vi "SourceDialog.vi"(8 "Error In":errorcluster, 11 "Source Configurations In":T1[](array[typedef])) -> (0 "Error Out":errorcluster, 2 "Cancelled?":bool, 3 "Source Configurations Out":T1[](array[typedef]))   [LabVIEW 2012]
uses:
  SourceConfiguration.ctl
  SourceFunction.ctl
  libs/LV-Utilities/LV-Utilities.lvlib
panel:
  in  "SMU B Auto Range Active?":bool=TRUE
  in  "SMU B Low Limit (V or A)":dbl format="%_4p"
  in  "SMU B High Limit (V or A)":dbl format="%_4p"
  in  "SMU B Active?":bool=TRUE
  in  "SMU B Level (V or A)":dbl format="%_4p"
  in  "SMU B Function":enum16{"Voltage", "Current"}(ring)
  in  "SMU A Auto Range Active?":bool=TRUE
  in  "SMU A Low Limit (V or A)":dbl format="%_4p"
  in  "SMU A High Limit (V or A)":dbl format="%_4p"
  in  "SMU A Active?":bool=TRUE
  in  "SMU A Level (V or A)":dbl format="%_4p"
  in  "SMU A Function":enum16{"Voltage", "Current"}(ring)
  in  "CANCEL":bool
  in  "DONE":bool
  # "SOURCE-MEASURE UNIT B"
  # "Range"
  # "Auto"
  # "Low Limit"
  # "High Limit"
  # "General"
  # "Active"
  # "Level"
  # "Function"
  # "SOURCE-MEASURE UNIT A"
  # "Range"
  # "Auto"
  # "Low Limit"
  # "High Limit"
  # "General"
  # "Active"
  # "Level"
  # "Function"
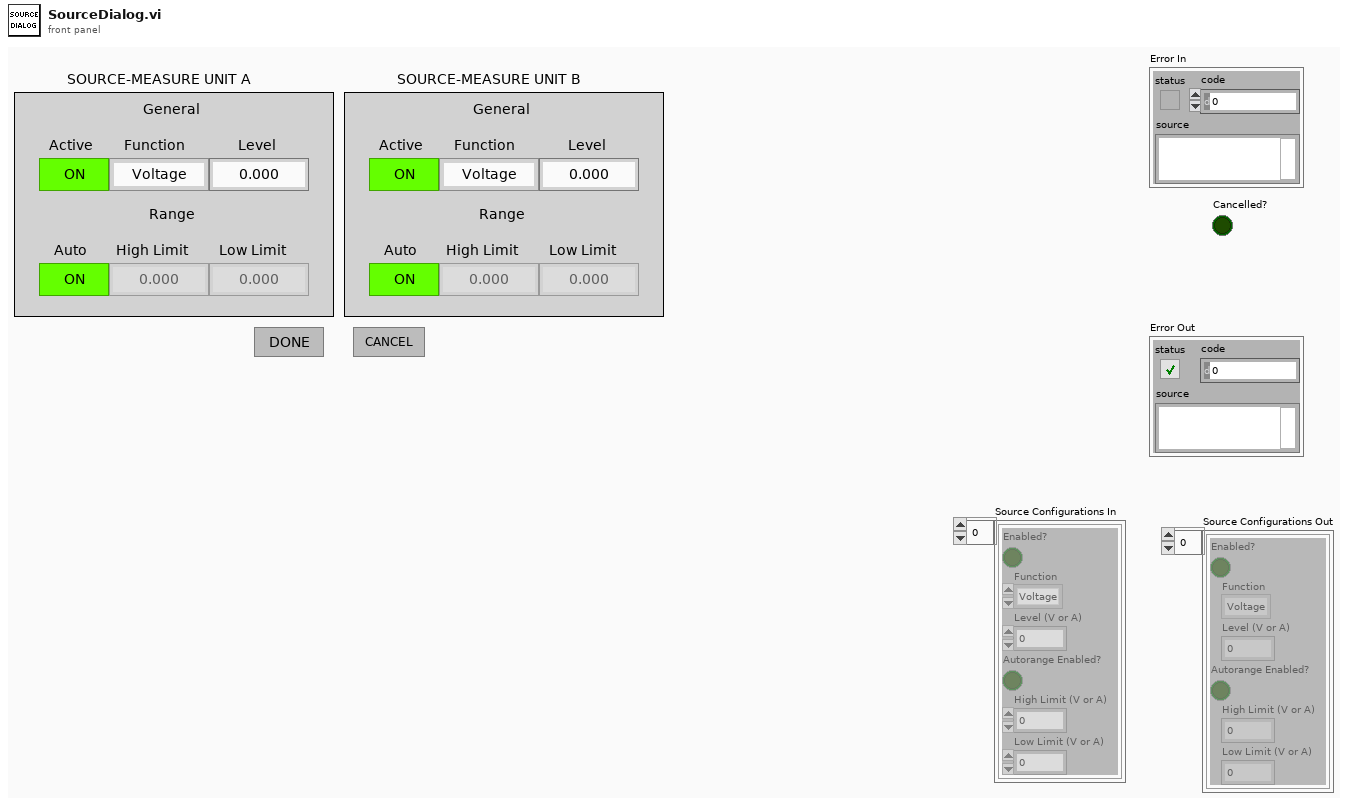
[diagram p1: front panel]
types:
  T1 = typedef "SourceConfiguration.ctl" = cluster{"Enabled?":bool, "Function":T2, "Level (V or A)":dbl, "Autorange Enabled?":bool, "High Limit (V or A)":dbl, "Low Limit (V or A)":dbl}
  T2 = typedef "SourceFunction.ctl" = enum16{"Voltage", "Current"}
  T3 = enum8{"Enabled", "Disabled", "Disabled and Grayed Out"}
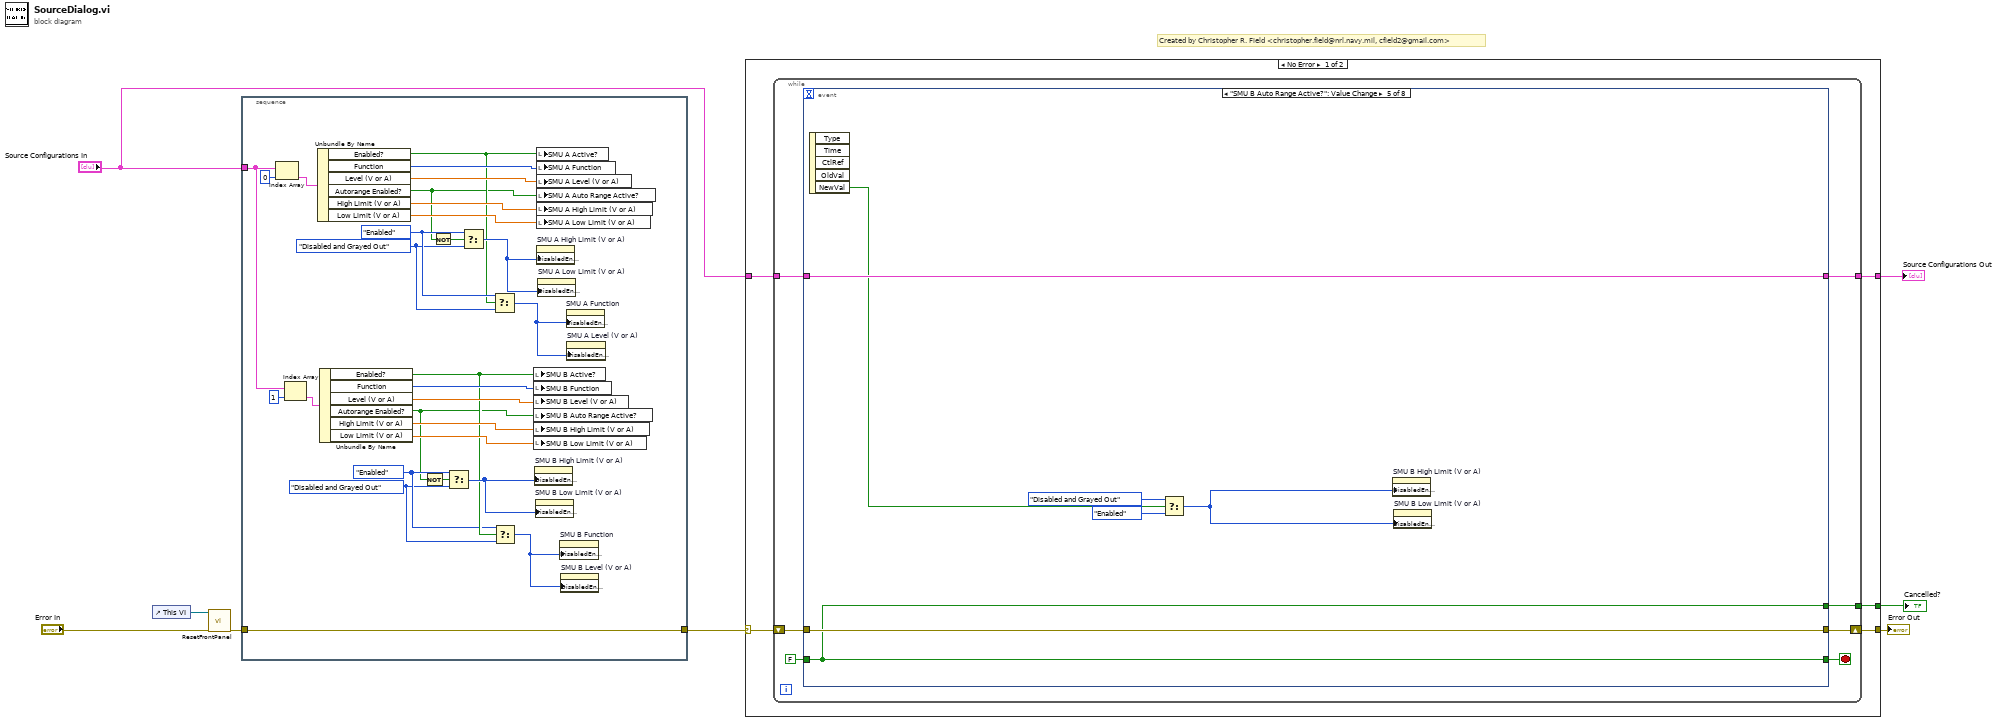
[diagram p0: block diagram]
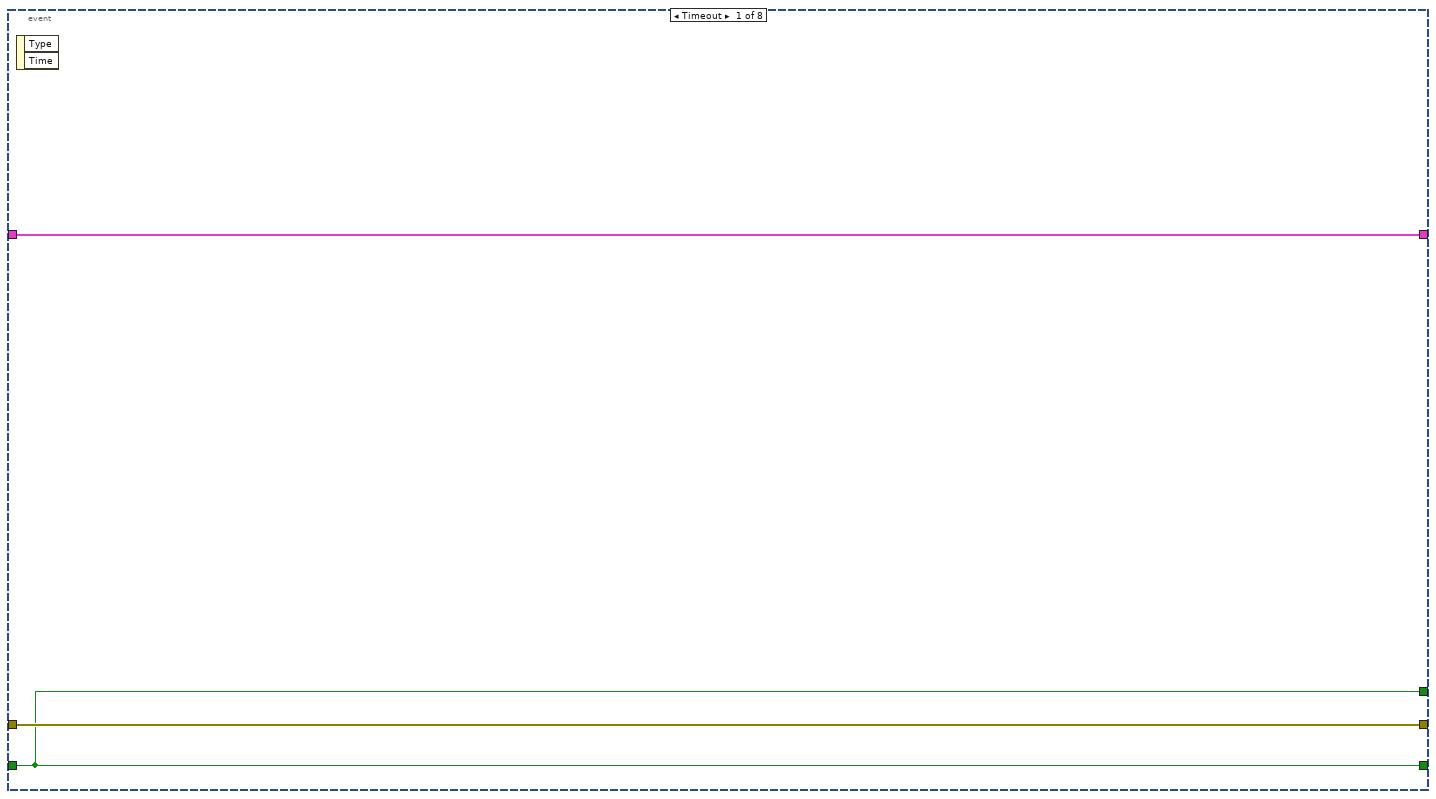
[diagram p2: hidden frame]
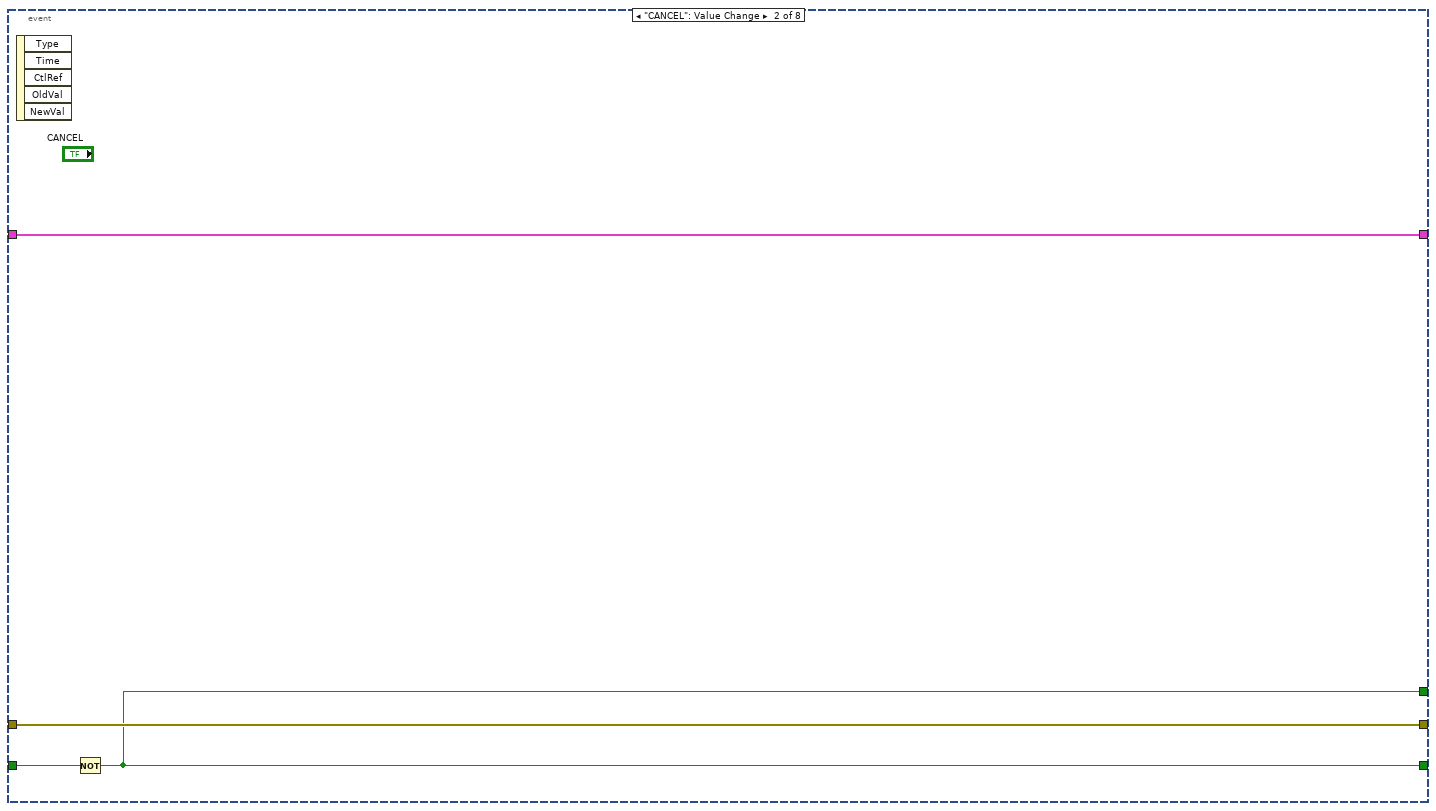
[diagram p3: hidden frame]
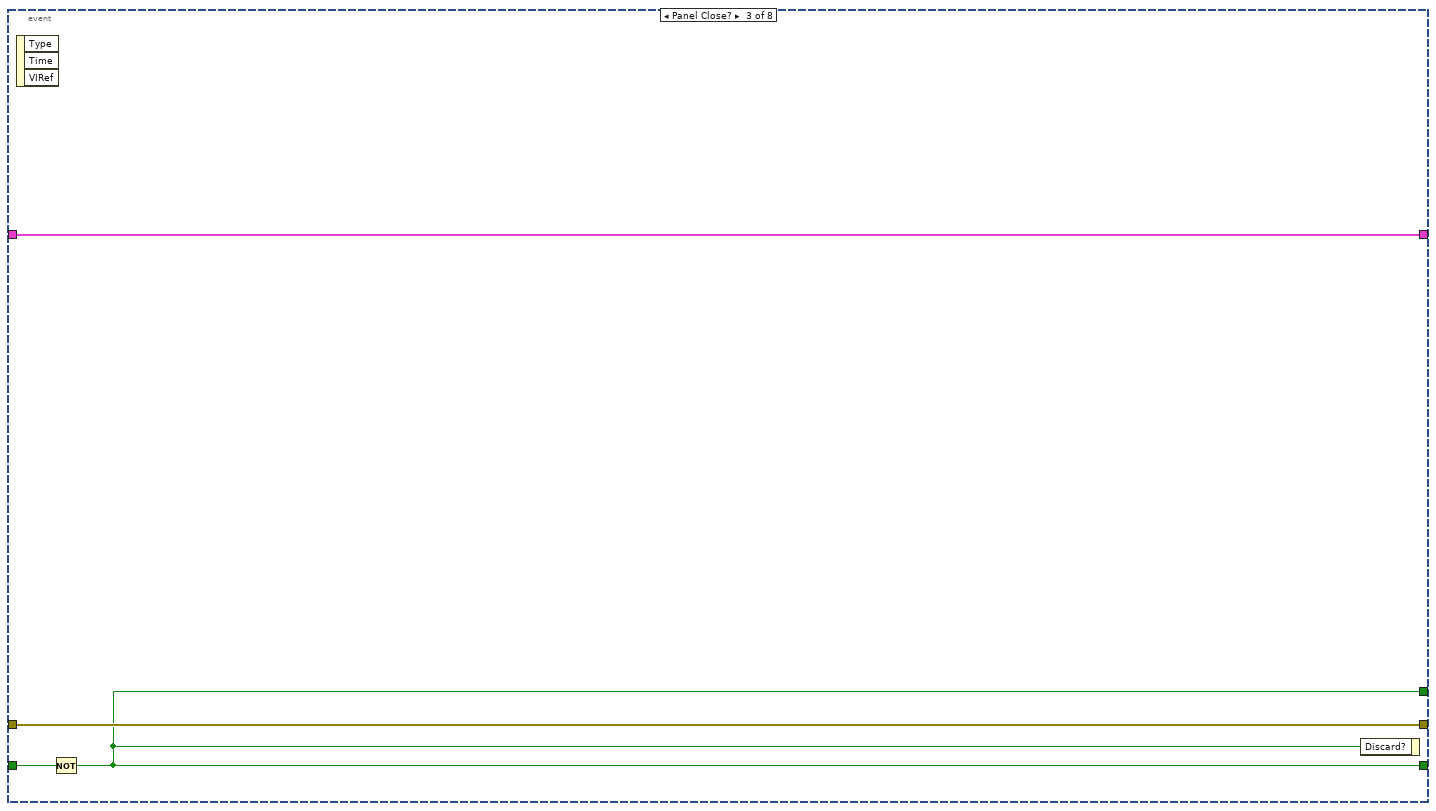
[diagram p4: hidden frame]
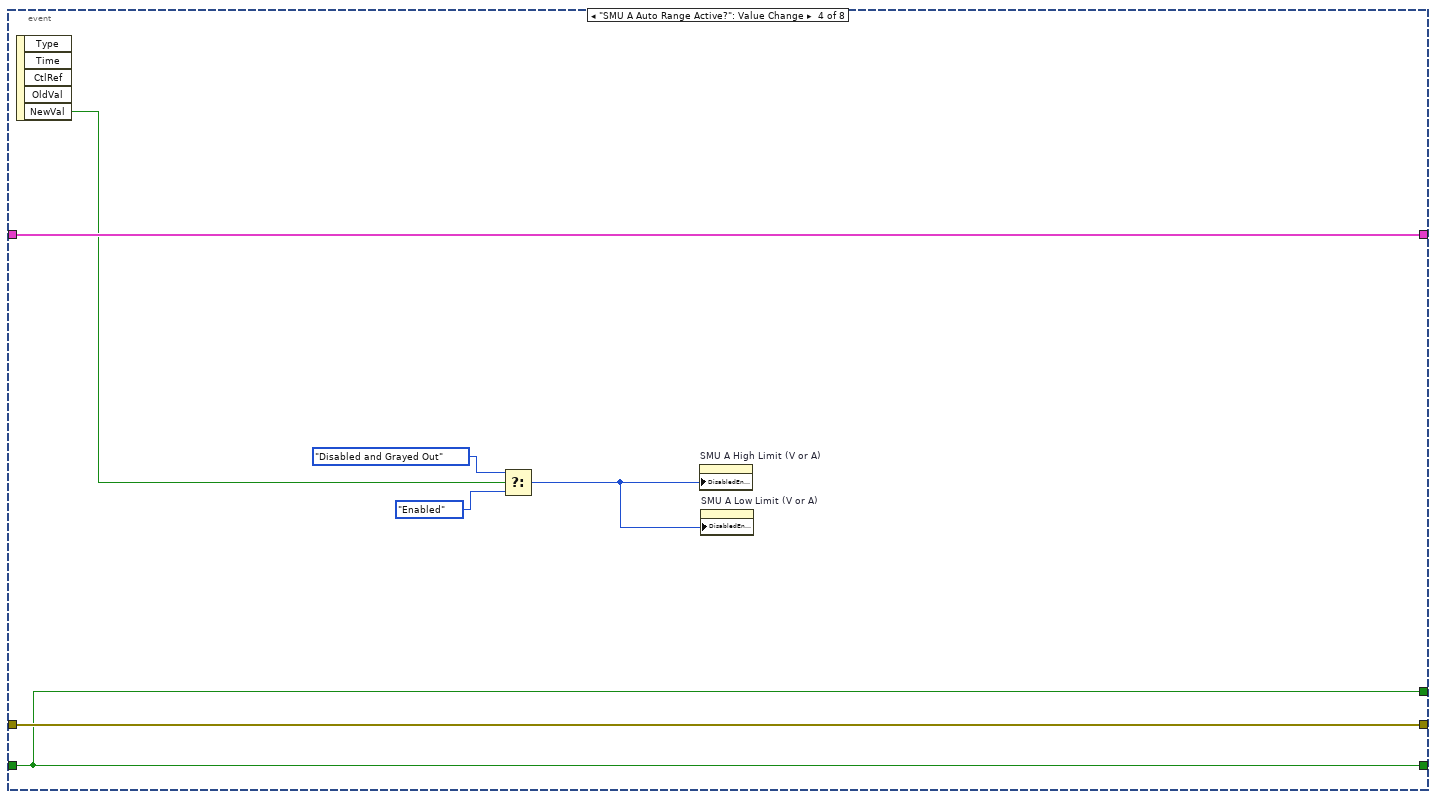
[diagram p5: hidden frame]
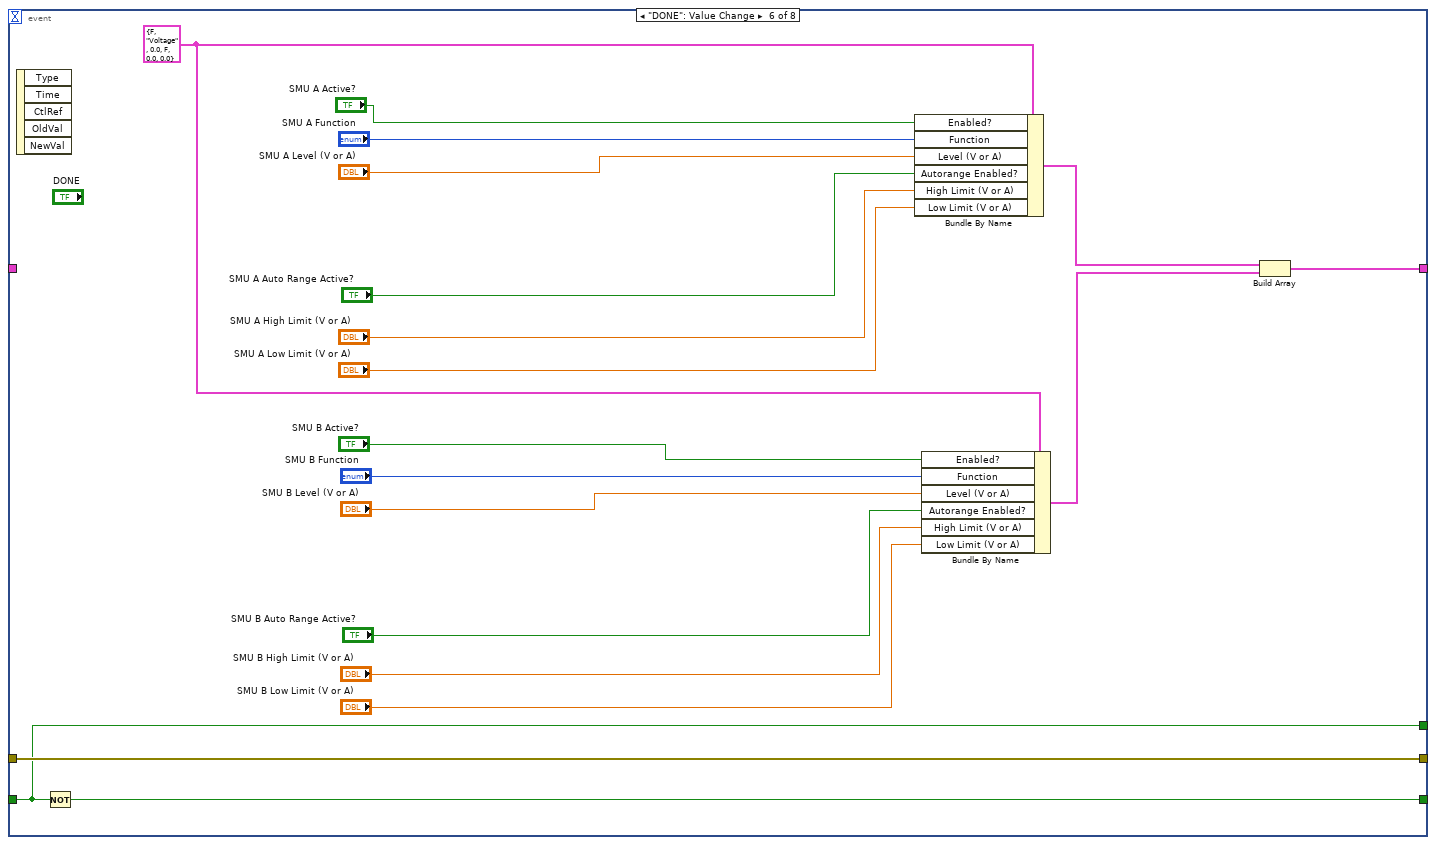
[diagram p6: hidden frame]
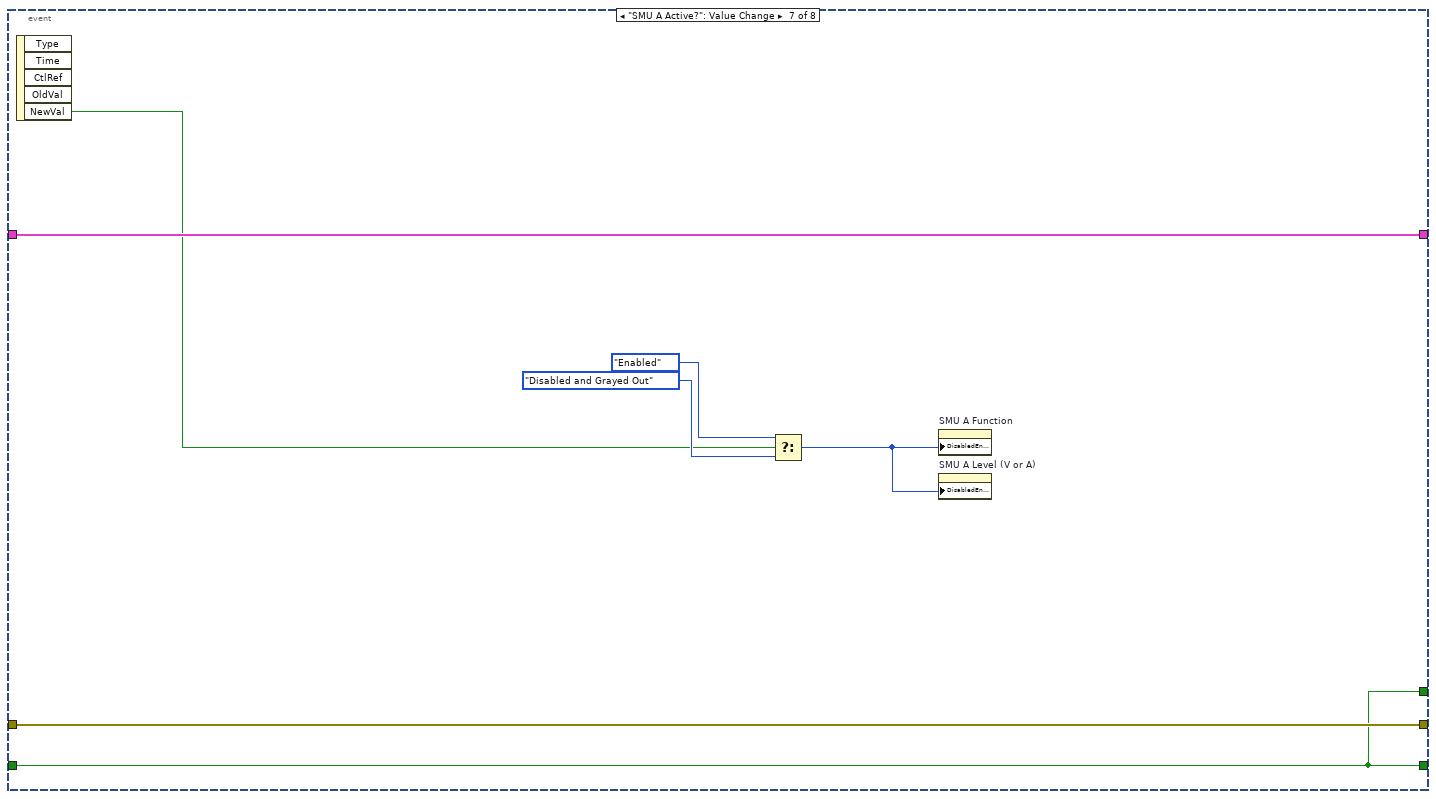
[diagram p7: hidden frame]
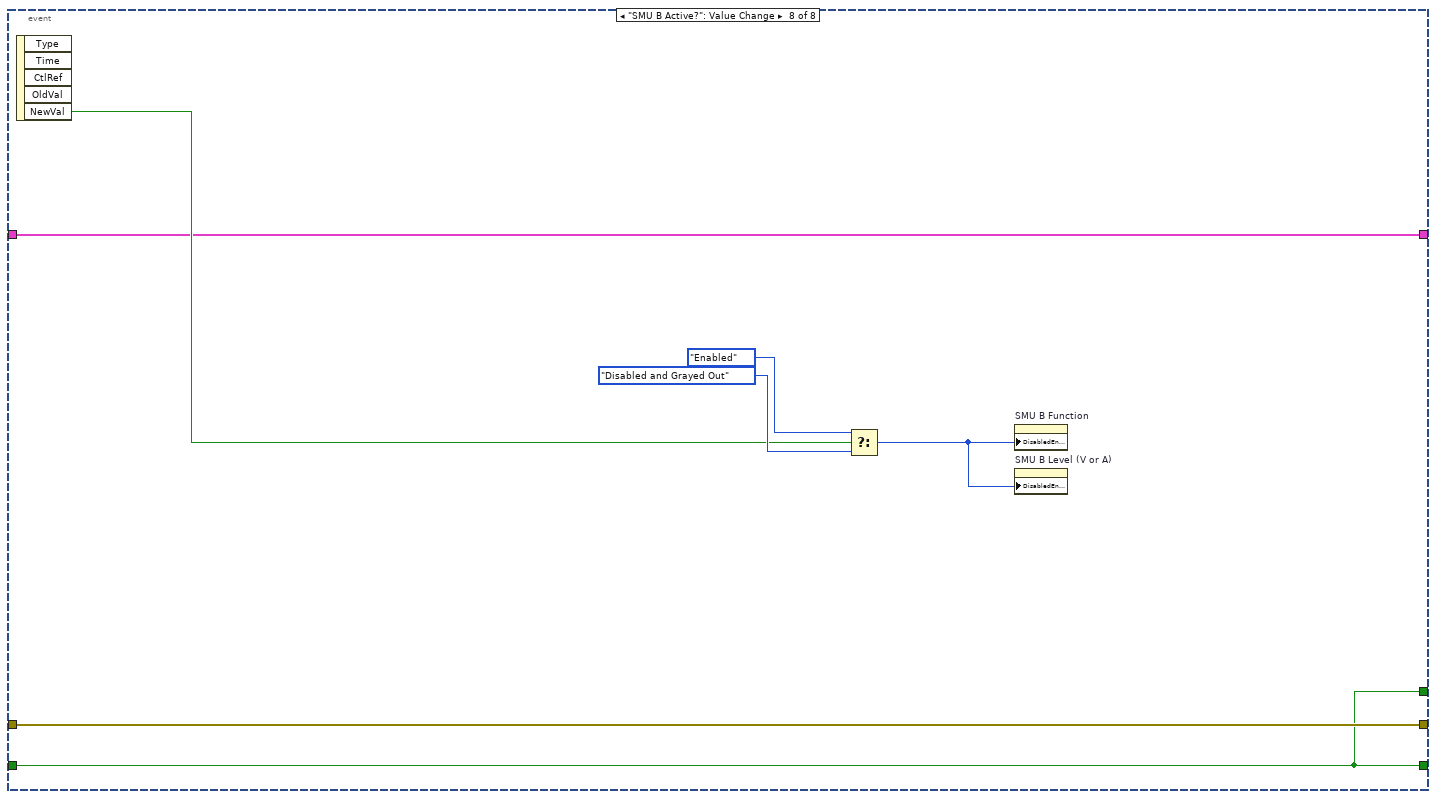
[diagram p8: hidden frame]
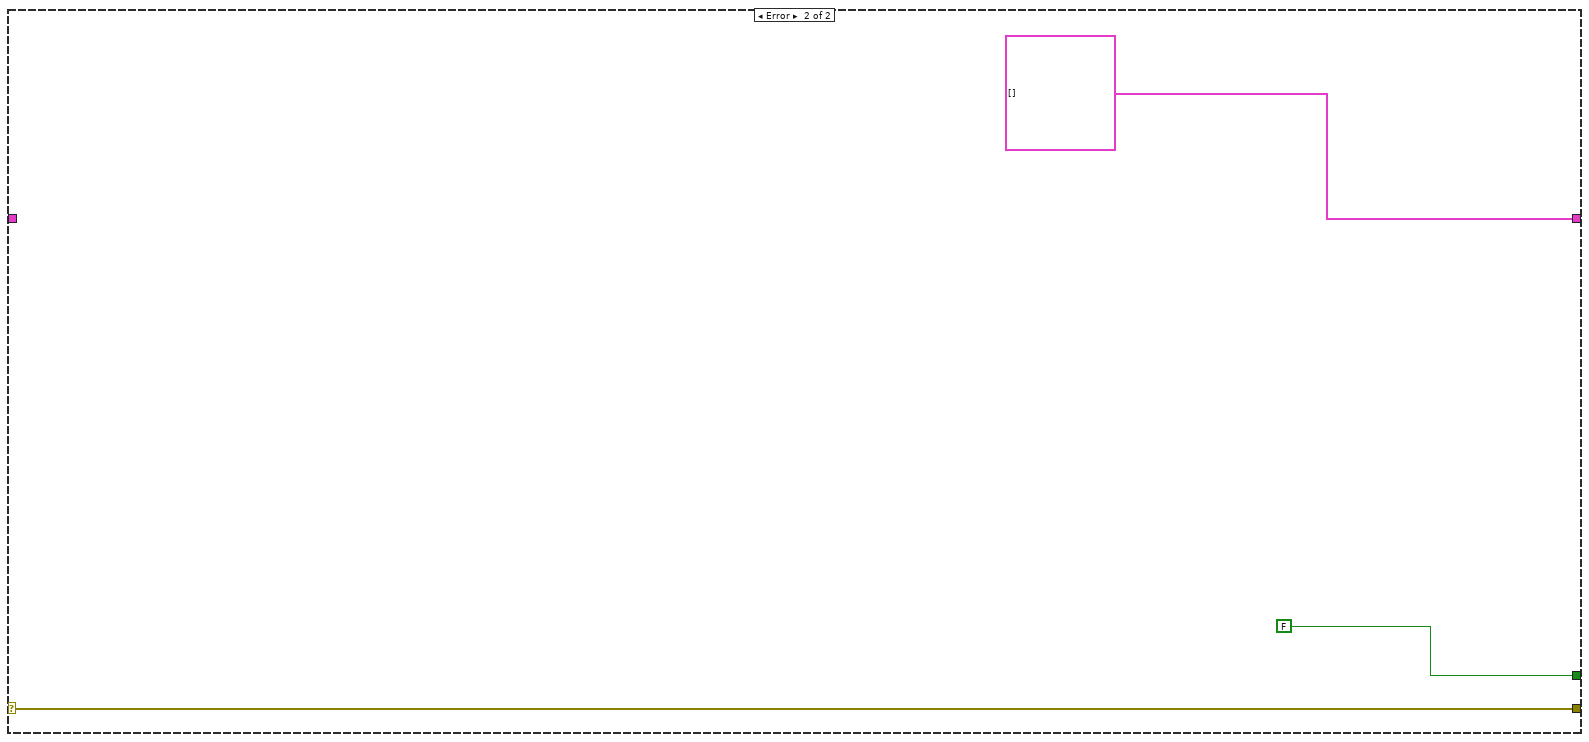
[diagram p9: hidden frame]
diagram:
  # "Created by Christopher R. Field <christopher.field@nrl.navy.mil, cfield2@gmail.com>"
  n1 = control-ref of="This VI"() -> (w1:refnum<vi>)
  n2 = call "ResetFrontPanel.vi"("Error In"="Error In", "VI Ref In"=w1) -> ("Error Out"=w4:errorcluster)  [unwired: 8 in, 1 out]
  n3 = stacked-sequence {
    tunnel: w4 -> [w36]
    tunnel: [w36] -> w3
    tunnel: "Source Configurations In" -> [w29]
    frame #0 {
      w18 = T3."Disabled and Grayed Out" ("f")
      w19 = T3."Enabled" ("Disabled")
      w13 = T3."Disabled and Grayed Out" ("f")
      w14 = T3."Enabled" ("Disabled")
      n4 = Index Array(array=w29, index=0) -> (element=w34:T1)
      n5 = Index Array(array=w29, index=1) -> (element=w27:T1)
      n6 = Unbundle By Name(w34) -> ("Enabled?"=w17:bool, "Function"=w33:T2, "Level (V or A)"=w32:dbl, "Autorange Enabled?"=w9:bool, "High Limit (V or A)"=w31:dbl, "Low Limit (V or A)"=w30:dbl)
      n7 = Unbundle By Name(w27) -> ("Enabled?"=w15:bool, "Function"=w26:T2, "Level (V or A)"=w25:dbl, "Autorange Enabled?"=w12:bool, "High Limit (V or A)"=w24:dbl, "Low Limit (V or A)"=w23:dbl)
      n8 = Not(x=w12) -> (.not. x?=w11:bool)
      n9 = Not(x=w9) -> (.not. x?=w10:bool)
      n10 = Select(t=w14, s=w11, f=w13) -> (s? t:f=w22:T3)
      n11 = Select(t=w19, s=w10, f=w18) -> (s? t:f=w21:T3)
      n12 = Select(t=w19, s=w17, f=w18) -> (s? t:f=w20:T3)
      n13 = Select(t=w14, s=w15, f=w13) -> (s? t:f=w16:T3)
      n14 = local write "SMU B Active?"(w15) -> ()
      n15 = local write "SMU B Function"(w26) -> ()
      n16 = local write "SMU B Level (V or A)"(w25) -> ()
      n17 = local write "SMU B Auto Range Active?"(w12) -> ()
      n18 = local write "SMU B High Limit (V or A)"(w24) -> ()
      n19 = local write "SMU B Low Limit (V or A)"(w23) -> ()
      n20 = property on="SMU B High Limit (V or A)" class="DigNum (strict)"("DisabledEnum"=w22) -> ()  [unwired: 2 in, 2 out]
      n21 = property on="SMU B Low Limit (V or A)" class="DigNum (strict)"("DisabledEnum"=w22) -> ()  [unwired: 2 in, 2 out]
      n22 = local write "SMU A Active?"(w17) -> ()
      n23 = local write "SMU A Function"(w33) -> ()
      n24 = local write "SMU A Level (V or A)"(w32) -> ()
      n25 = local write "SMU A Auto Range Active?"(w9) -> ()
      n26 = local write "SMU A High Limit (V or A)"(w31) -> ()
      n27 = local write "SMU A Low Limit (V or A)"(w30) -> ()
      n28 = property on="SMU A High Limit (V or A)" class="DigNum (strict)"("DisabledEnum"=w21) -> ()  [unwired: 2 in, 2 out]
      n29 = property on="SMU A Low Limit (V or A)" class="DigNum (strict)"("DisabledEnum"=w21) -> ()  [unwired: 2 in, 2 out]
      n30 = property on="SMU B Function" class="Enum (strict)"("DisabledEnum"=w16) -> ()  [unwired: 2 in, 2 out]
      n31 = property on="SMU B Level (V or A)" class="DigNum (strict)"("DisabledEnum"=w16) -> ()  [unwired: 2 in, 2 out]
      n32 = property on="SMU A Function" class="Enum (strict)"("DisabledEnum"=w20) -> ()  [unwired: 2 in, 2 out]
      n33 = property on="SMU A Level (V or A)" class="DigNum (strict)"("DisabledEnum"=w20) -> ()  [unwired: 2 in, 2 out]
    }
  }
  n34 = case shown="No Error" w3 {
    selector: w3 -> [w40 w109]
    tunnel: [w41 w109] -> w7
    tunnel: [w39 FALSE] -> w6
    tunnel: [w38 T1[] []] -> w5
    tunnel: "Source Configurations In" -> [w37 _]
    frame No Error {
      n35 = while {
        shift-right: [w46] -> w41
        shift-left: w40 -> [w45]
        tunnel: [w44] -> w39
        tunnel: [w43] -> w38
        tunnel: w37 -> [w42]
        stop <- w47 stop-if-true
        n36 = event shown="[4] \"SMU B Auto Range Active?\": Value Change" {
          selector: _ -> [_ _ _ _ _ _ _ _]
          dyn-events: _ -> [_ _ _ _ _ _ _ _]
          timeout: _ -> [_ _ _ _ _ _ _ _]
          tunnel: FALSE -> [w50 w55 w59 w65 w72 w90 w97 w100]
          tunnel: [w50 w53 w57 w65 w72 w92 w97 w100] -> w47
          tunnel: w45 -> [w51 w54 w58 w66 w73 w91 w98 w101]
          tunnel: [w51 w54 w58 w66 w73 w91 w98 w101] -> w46
          tunnel: [w50 w53 w57 w65 w72 w90 w97 w100] -> w44
          tunnel: [w49 w52 w56 w64 w71 w78 w99 w102] -> w43
          tunnel: w42 -> [w49 w52 w56 w64 w71 _ w99 w102]
          event Timeout {
            n37 = event-data() -> ()  [unwired: 1 in, 2 out]
          }
          event "CANCEL": Value Change {
            n38 = event-data() -> ()  [unwired: 1 in, 5 out]
            n39 = Not(x=w55) -> (.not. x?=w53:bool)
          }
          event Panel Close? {
            n40 = event-data() -> ()  [unwired: 1 in, 3 out]
            n41 = Not(x=w59) -> (.not. x?=w57:bool)
            n42 = event-data("Discard?"=w57) -> ()  [unwired: 1 in, 1 out]
          }
          event "SMU A Auto Range Active?": Value Change {
            n43 = event-data() -> ("NewVal"=w63:bool)  [unwired: 1 in, 4 out]
            n44 = Select(t=T3."Disabled and Grayed Out" ("Disabled"), s=w63, f=T3."Enabled" ("Disabled")) -> (s? t:f=w60:T3)
            n45 = property on="SMU A High Limit (V or A)" class="DigNum (strict)"("DisabledEnum"=w60) -> ()  [unwired: 2 in, 2 out]
            n46 = property on="SMU A Low Limit (V or A)" class="DigNum (strict)"("DisabledEnum"=w60) -> ()  [unwired: 2 in, 2 out]
          }
          event "SMU B Auto Range Active?": Value Change {
            n47 = event-data() -> ("NewVal"=w69:bool)  [unwired: 1 in, 4 out]
            n48 = Select(t=T3."Disabled and Grayed Out" ("Disabled"), s=w69, f=T3."Enabled") -> (s? t:f=w67:T3)
            n49 = property on="SMU B High Limit (V or A)" class="DigNum (strict)"("DisabledEnum"=w67) -> ()  [unwired: 2 in, 2 out]
            n50 = property on="SMU B Low Limit (V or A)" class="DigNum (strict)"("DisabledEnum"=w67) -> ()  [unwired: 2 in, 2 out]
          }
          event "DONE": Value Change {
            w84 = T1 {"Enabled?"=FALSE, "Function"=enum."Voltage", "Level (V or A)"=0.0, "Autorange Enabled?"=FALSE, "High Limit (V or A)"=0.0, "Low Limit (V or A)"=0.0} ("Source Configuration")
            n51 = event-data() -> ()  [unwired: 1 in, 5 out]
            n52 = Not(x=w90) -> (.not. x?=w92:bool)
            n53 = Bundle By Name(cluster=w84, "Enabled?"="SMU A Active?", "Function"="SMU A Function", "Level (V or A)"="SMU A Level (V or A)", "Autorange Enabled?"="SMU A Auto Range Active?", "High Limit (V or A)"="SMU A High Limit (V or A)", "Low Limit (V or A)"="SMU A Low Limit (V or A)") -> (w80:T1)
            n54 = Bundle By Name(cluster=w84, "Enabled?"="SMU B Active?", "Function"="SMU B Function", "Level (V or A)"="SMU B Level (V or A)", "Autorange Enabled?"="SMU B Auto Range Active?", "High Limit (V or A)"="SMU B High Limit (V or A)", "Low Limit (V or A)"="SMU B Low Limit (V or A)") -> (w79:T1)
            n55 = Build Array(w80, w79) -> (w78:T1[])
          }
          event "SMU A Active?": Value Change {
            n56 = event-data() -> ("NewVal"=w93:bool)  [unwired: 1 in, 4 out]
            n57 = Select(t=T3."Enabled" ("Disabled"), s=w93, f=T3."Disabled and Grayed Out" ("Disabled")) -> (s? t:f=w94:T3)
            n58 = property on="SMU A Function" class="Enum (strict)"("DisabledEnum"=w94) -> ()  [unwired: 2 in, 2 out]
            n59 = property on="SMU A Level (V or A)" class="DigNum (strict)"("DisabledEnum"=w94) -> ()  [unwired: 2 in, 2 out]
          }
          event "SMU B Active?": Value Change {
            n60 = event-data() -> ("NewVal"=w103:bool)  [unwired: 1 in, 4 out]
            n61 = Select(t=T3."Enabled" ("Disabled"), s=w103, f=T3."Disabled and Grayed Out" ("Disabled")) -> (s? t:f=w104:T3)
            n62 = property on="SMU B Function" class="Enum (strict)"("DisabledEnum"=w104) -> ()  [unwired: 2 in, 2 out]
            n63 = property on="SMU B Level (V or A)" class="DigNum (strict)"("DisabledEnum"=w104) -> ()  [unwired: 2 in, 2 out]
          }
        }
      }
    }
    frame Error {
    }
  }
  "Error Out" <- w7
  "Cancelled?" <- w6
  "Source Configurations Out" <- w5
